vi "open.vi"(8 "error in (no error)":errorcluster, 10 "index":u32) -> (0 "error out":errorcluster, 3 "DevRefnum":u64)   [LabVIEW 2013, in "rtlsdr.lvlib"]
doc: "RTLSDR_API int rtlsdr_open(rtlsdr_dev_t **dev, uint32_t index);"
uses:
  <instrlib>/rtlsdr/rtlsdr.lvlib
  <instrlib>/rtlsdr/VIs/rtlsdr.dll
panel:
  in  "DevRefnum":u64
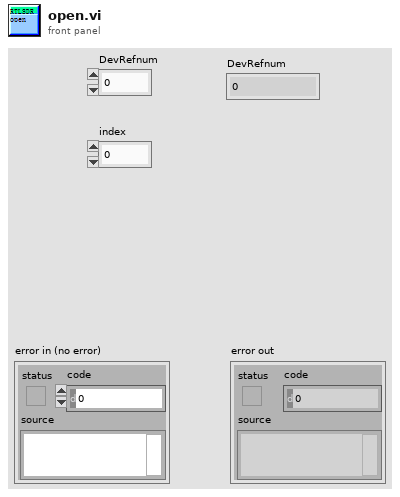
[diagram p1: front panel]
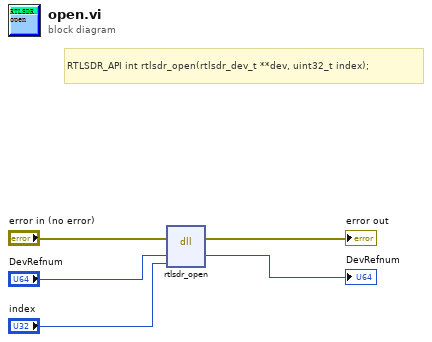
[diagram p0: block diagram]
diagram:
  # "RTLSDR_API int rtlsdr_open(rtlsdr_dev_t **dev, uint32_t index);"
  n1 = dll-call lib="C:/Program Files (x86)/National Instruments/LabVIEW 2013/instr.lib/rtlsdr/VIs/rtlsdr.*" fn="rtlsdr_open"(error in="error in (no error)", "DevRefnum"="DevRefnum", "index"="index") -> (error out=→"error out":errorcluster, "DevRefnum"=→"DevRefnum":u64)  [unwired: 4 in, 1 out]
